vi "Reset.vi"(8 "error in (no error)":errorcluster, 10 "Mouse In":refnum<class "Mouse.lvclass">, 11 "Maze in":refnum<class "Maze.lvclass">) -> (0 "error out":errorcluster, 2 "Mouse":refnum<class "Mouse.lvclass">, 3 "Maze out":refnum<class "Maze.lvclass">)   [LabVIEW 2020, in "Maze.lvlib" / "Maze.lvclass"]
uses:
  Maze.lvclass
  Mouse/Mouse.lvclass
  Direction.ctl
  Maze.lvclass/Maze.ctl
  Maze.lvlib
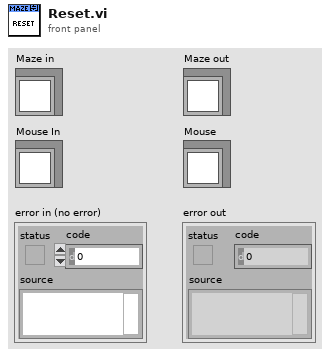
[diagram p1: front panel]
types:
  T1 = typedef "Maze.lvlib/Direction.ctl" = enum8{"East", "North", "West", "South"}
  T2 = typedef "Maze.lvlib/Position.ctl" = cluster{"S":i32, "E":i32}
  T3 = typedef "Maze.lvlib/Adjacency.ctl" = cluster{"E":bool, "N":bool, "W":bool, "S":bool, "Goal":bool, "Start":bool}
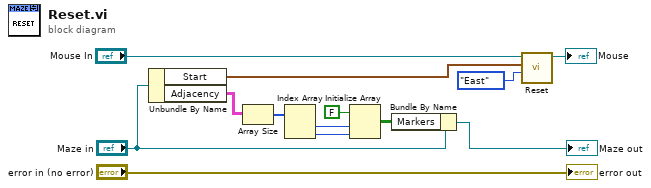
[diagram p0: block diagram]
diagram:
  n1 = Unbundle By Name("Maze in") -> ("Start"=w8:T2, "Adjacency"=w7:T3[][])
  n2 = Array Size(array=w7) -> (size(s)=w6:i32[])
  n3 = Index Array(array=w6) -> (element #1=w4:i32, element #2=w3:i32)  [unwired: 2 in]
  n4 = Initialize Array(FALSE, w4, w3) -> (w1:bool[][])
  n5 = Bundle By Name(cluster="Maze in", "Markers"=w1) -> (→"Maze out":refnum<class "Maze.lvclass">)
  n6 = call "Reset.vi"("Direction"=Direction."East", "Position"=w8, "Mouse in"="Mouse In") -> ("Mouse out"=→"Mouse":refnum<class "Mouse.lvclass">)  [unwired: 7 in, 1 out]
  "error out" <- "error in (no error)"
